vi "Setup_acquire_test.vi"() -> ()   [LabVIEW 2010]
uses:
  <userlib>/BIAS2/subvis/ROI_rect.ctl
  <userlib>/BIAS2/subvis/ExposureSettings.ctl
  <vilib>/Utility/error.llb/DialogType.ctl
  <userlib>/BIAS2/classes/CameraBase/CameraBase.lvclass
panel:
  out "error out":errorcluster
  out "Intensity Graph":u16[][](graph)
  out "image_data":u16[][][](array[numeric])
  out "acquiring":bool caption="Acquiring"
  in  "binning":cluster{"x":u8, "y":u8}={"x"=1, "y"=1}
  in  "Timeout":u32=500
  out "roi_capture":T1={"left"=686, "top"=399, "right"=1281, "bottom"=1004}
  out "image_size":i32[](array[numeric])
  out "attribs":variant[](array[variant])
  out "roi_sensor":T1={"left"=0, "top"=0, "right"=1936, "bottom"=1456} caption="camera size"
  in  "exposure":sgl=10.0 caption="exposure (ms)"
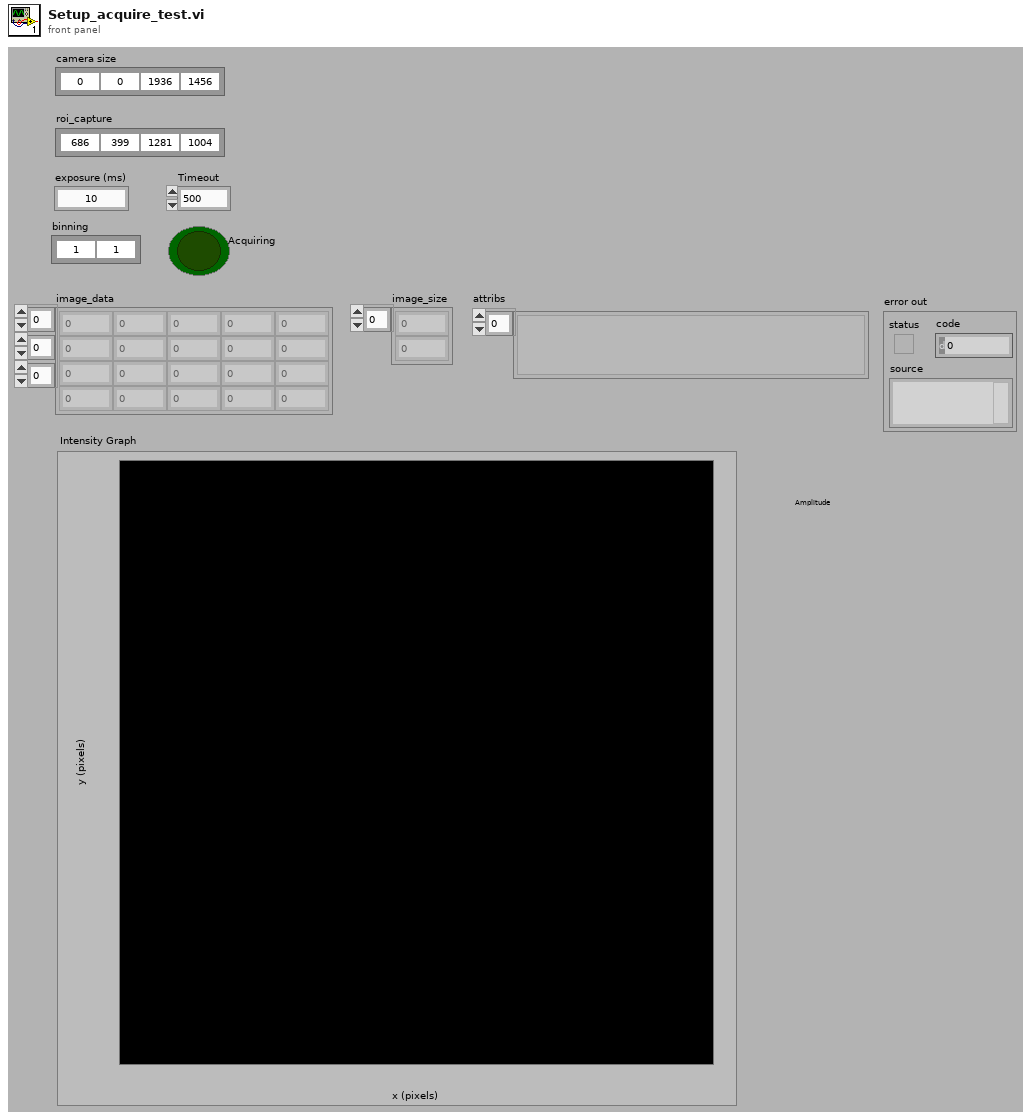
[diagram p1: front panel]
types:
  T1 = typedef "ROI_rect.ctl" = cluster{"left":i32, "top":i32, "right":i32, "bottom":i32}
  T2 = typedef "DialogType.ctl" = u16
  T3 = typedef "ExposureSettings.ctl" = cluster{"exposure":dbl, "external":bool, "roi":T1, "frames":i32, "binning":cluster{"x":u8, "y":u8}}
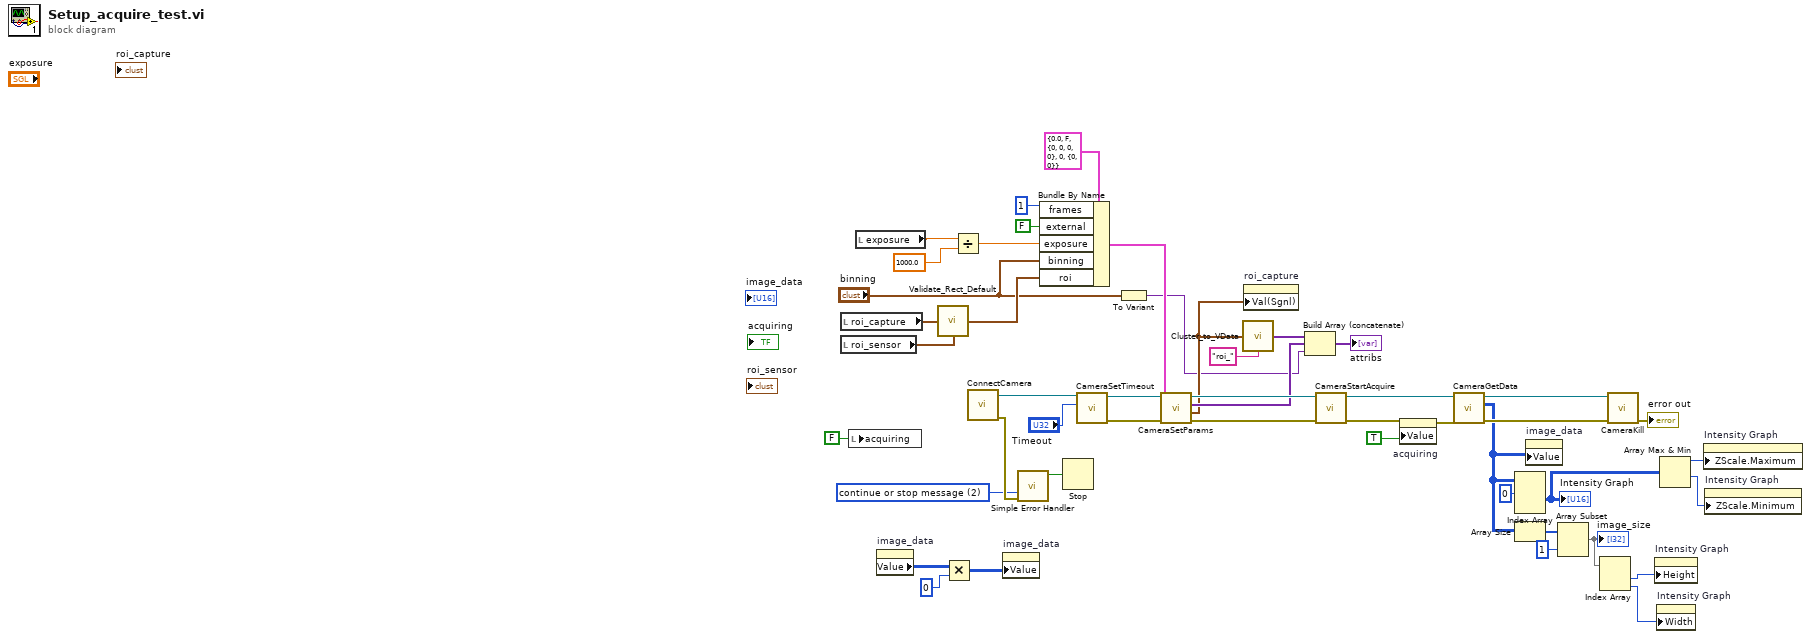
[diagram p0: block diagram]
diagram:
  w17 = T2 2 items=["no dialog", "OK message", "continue or stop message", "OK message + warnings", "continue/stop + warnings"] ("type of dialog (OK msg:1)")
  n1 = local read "roi_capture"() -> (w44:T1)
  n2 = local read "roi_sensor"() -> (w41:T1)
  n3 = local write "acquiring"(FALSE ("acquiring")) -> ()
  n4 = local read "exposure"() -> (w47:sgl)
  n5 = property on="image_data" class="Arr (strict)"() -> ("Value"=w12:u16[][][])  [unwired: 2 in, 2 out]
  n6 = call <userlib>:"Validate_Rect_Default.vi"("rect"=w44, "default"=w41) -> ("out"=w36:T1)
  n7 = Multiply(x=w12, y=0 ("index")) -> (x*y=w10:i32[][][])
  n8 = Divide(x=w47, y=sgl 1000.0) -> (x/y=w43:sgl)
  n9 = call <userlib>:"ConnectCamera.vi"() -> ("error out"=w19:errorcluster, "camera"=w14:refnum<class "CameraBase.lvclass">)  [unwired: 3 in, 5 out]
  n10 = property on="image_data" class="Arr (strict)"("Value"=w10) -> ()  [unwired: 2 in, 2 out]
  n11 = call <vilib>:"Simple Error Handler.vi"("type of dialog (OK msg:1)"=w17, "error in (no error)"=w19) -> ("error?"=w18:bool)  [unwired: 3 in, 4 out]
  n12 = Bundle By Name(cluster=T3 {"exposure"=0.0, "external"=FALSE, "roi"={"left"=0, "top"=0, "right"=0, "bottom"=0}, "frames"=0, "binning"={"x"=0, "y"=0}} ("settings"), "frames"=1, "external"=FALSE, "exposure"=w43, "binning"="binning", "roi"=w36) -> (w42:T3)
  n13 = Stop(stop? (T)=w18) -> ()
  n14 = call-dynamic "CameraSetTimeout.vi"("Timeout"="Timeout", "CameraBase in"=w14) -> ("error out"=w31:errorcluster, "CameraBase out"=w38:refnum<class "CameraBase.lvclass">)  [unwired: 7 in, 1 out]
  n15 = To Variant(anything="binning") -> (Variant=w33:variant)
  n16 = call-dynamic "CameraSetParams.vi"("error in (no error)"=w31, "settings"=w42, "CameraBase in"=w38) -> ("error out"=w30:errorcluster, "roi_out"=w37:T1, "attributes"=w39:variant[], "CameraBase out"=w40:refnum<class "CameraBase.lvclass">)  [unwired: 5 in]
  n17 = call <userlib>:"Cluster_to_VData.vi"("cluster"=w37, "prefix"="roi_") -> ("vdata"=w28:variant[])
  n18 = property on="roi_capture" class="Clust (strict)"("Val(Sgnl)"=w37) -> ()  [unwired: 2 in, 2 out]
  n19 = Build Array (concatenate)(w28, w39, w33) -> (→"attribs":variant[])
  n20 = call-dynamic "CameraStartAcquire.vi"("error in (no error)"=w30, "CameraBase in"=w40) -> ("error out"=w25:errorcluster, "CameraBase out"=w23:refnum<class "CameraBase.lvclass">)  [unwired: 8 in]
  n21 = property on="acquiring" class="Bool (strict)"(error in=w25, "Value"=TRUE ("acquiring")) -> (error out=w24:errorcluster)  [unwired: 1 in, 1 out]
  n22 = call-dynamic "CameraGetData.vi"("error in (no error)"=w24, "CameraBase in"=w23) -> ("error out"=w15:errorcluster, "image_data"=w9:u16[][][], "CameraBase out"=w16:refnum<class "CameraBase.lvclass">)  [unwired: 7 in]
  n23 = Index Array(array=w9, index (dim 0)=0 ("index (page)")) -> (element=w5:u16[][])  [unwired: 2 in]
  "Intensity Graph" <- w5
  n24 = Array Size(array=w9) -> (size(s)=w35:i32[])
  n25 = property on="image_data" class="Arr (strict)"("Value"=w9) -> ()  [unwired: 2 in, 2 out]
  n26 = Array Subset(array=w35, index=1) -> (w7:i32[])  [unwired: 1 in]
  "image_size" <- w7
  n27 = Index Array(array=w7) -> (element #1=w4:i32, element #2=w3:i32)  [unwired: 2 in]
  n28 = call-dynamic "CameraKill.vi"("error in (no error)"=w15, "CameraBase in"=w16) -> ("error out"=→"error out":errorcluster)  [unwired: 8 in, 1 out]
  n29 = property on="Intensity Graph" class="IntGraph (strict)"("Height"=w4) -> ()  [unwired: 2 in, 2 out]
  n30 = property on="Intensity Graph" class="IntGraph (strict)"("Width"=w3) -> ()  [unwired: 2 in, 2 out]
  n31 = Array Max & Min(array=w5) -> (max value=w2:u16, min value=w1:u16)  [unwired: 2 out]
  n32 = property on="Intensity Graph" class="IntGraph (strict)"("ZScale.Maximum"=w2) -> ()  [unwired: 2 in, 2 out]
  n33 = property on="Intensity Graph" class="IntGraph (strict)"("ZScale.Minimum"=w1) -> ()  [unwired: 2 in, 2 out]
